vi "getParent.vi"(0 "reference":refnum<class "AbstractNode.lvclass">, 5 "error in (no error)":errorcluster) -> (14 "reference out":refnum<class "AbstractNode.lvclass">, 15 "parentNode":refnum<class "AbstractNode.lvclass">, 16 "ValidParent":bool, 17 "Ref":u32, 19 "error out":errorcluster)   [LabVIEW 2012, in "AbstractNode.lvclass"]
doc: "public Node getParent()"
uses:
  <resource>/Framework/Providers/Open_GDS/UML/AbstractNode_class/AbstractNode.lvclass
  <resource>/Framework/Providers/Open_GDS/UML/AbstractNode_class/AbstractNode.lvclass/AbstractNode.ctl
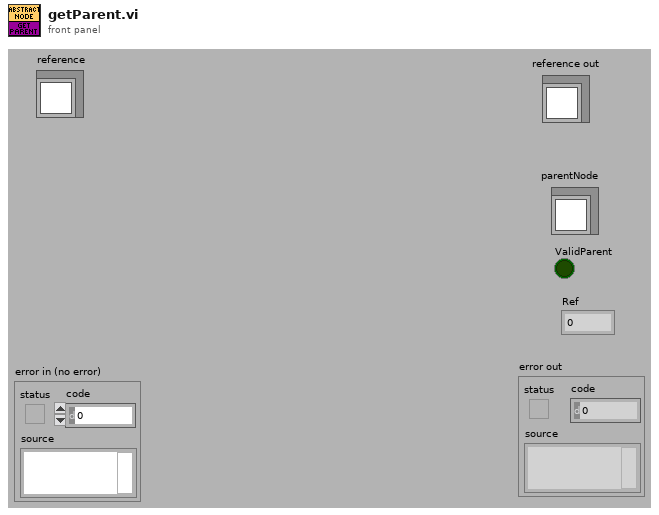
[diagram p1: front panel]
types:
  T1 = typedef "AbstractNode.lvclass/ObjectAttributes.ctl" = cluster{"parent":refnum<class "AbstractNode.lvclass">, "children":refnum<class "AbstractNode.lvclass">[], "Hidden":bool}
  T2 = typedef "AbstractNode.lvclass/ObjectReference.ctl" = refnum<k1>
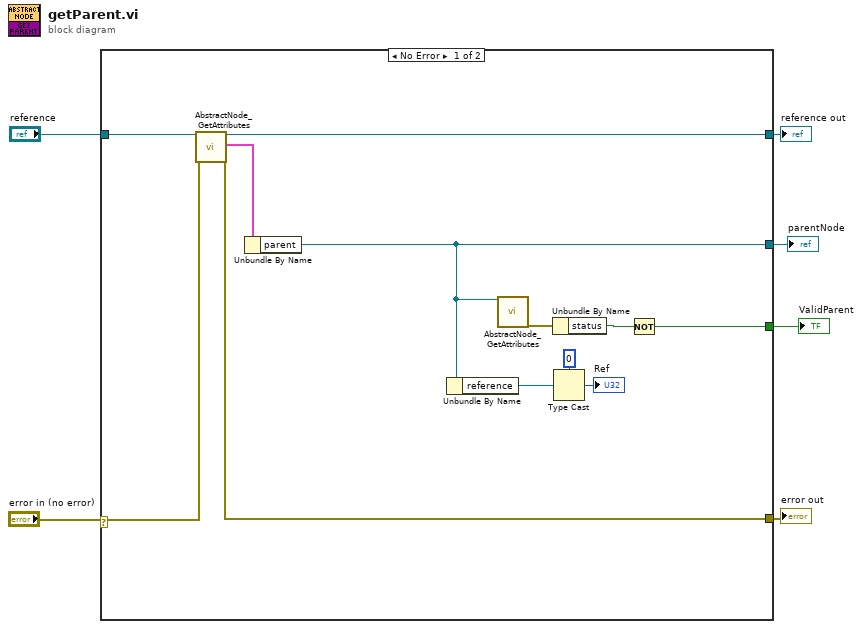
[diagram p0: block diagram]
diagram:
  n1 = case shown="No Error" "error in (no error)" {
    selector: "error in (no error)" -> [w15 w19]
    tunnel: "reference" -> [w18 w20]
    tunnel: [w17 w19] -> w5
    tunnel: [w16 w20] -> w4
    tunnel: [w10 _] -> w2
    tunnel: [w11 _] -> w1
    frame No Error {
      n2 = call <resource>:"AbstractNode_GetAttributes.vi"("reference in"=w18, "error in (no error)"=w15) -> ("reference out"=w16:refnum<class "AbstractNode.lvclass">, "Attributes"=w14:T1, "error out"=w17:errorcluster)  [unwired: 15 out]
      n3 = Unbundle By Name(w14) -> ("parent"=w10:refnum<class "AbstractNode.lvclass">)
      n4 = Unbundle By Name(w10) -> ("reference"=w8:T2)
      n5 = call <resource>:"AbstractNode_GetAttributes.vi"("reference in"=w10) -> ("error out"=w13:errorcluster)  [unwired: 1 in, 17 out]
      n6 = Unbundle By Name(w13) -> ("status"=w12:bool)
      n7 = Type Cast(type=u32 0, x=w8) -> (*(type *) &x=→"Ref":u32)
      n8 = Not(x=w12) -> (.not. x?=w11:bool)
    }
    frame Error {
    }
  }
  "reference out" <- w4
  "error out" <- w5
  "parentNode" <- w2
  "ValidParent" <- w1
